vi "Read Menu Name.vi"(8 "error in":errorcluster, 11 "Engine Parent in":refnum<class "Engine Parent Editor Node.lvclass">) -> (0 "error out":errorcluster, 2 "Name":string, 3 "Engine Parent out":refnum<class "Engine Parent Editor Node.lvclass">)   [LabVIEW 2013, in "PL Framework Configuration Tool.lvlib" / "Engine Parent Editor Node.lvclass"]
uses:
  Engine Parent Editor Node.lvclass
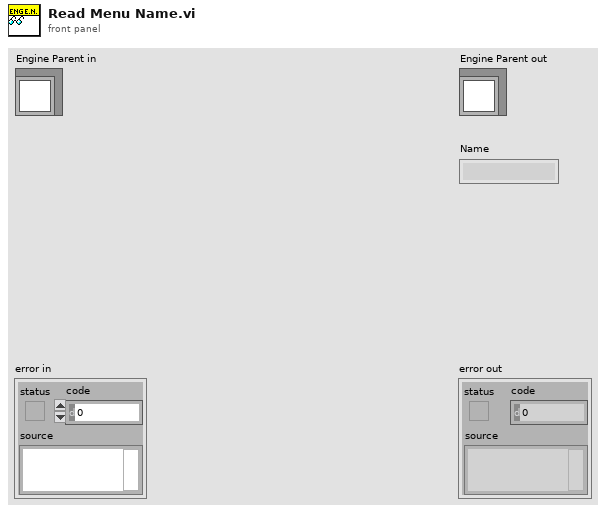
[diagram p1: front panel]
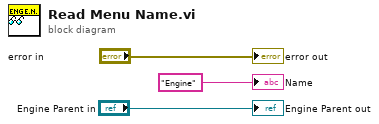
[diagram p0: block diagram]
diagram:
  "error out" <- "error in"
  "Engine Parent out" <- "Engine Parent in"
  "Name" <- "Engine" ("Name")
